vi "testWriteFileStylesheetAbsUrlHeaderPresent.vi"(8 "error in (no error)":errorcluster, 11 "TestCase in":refnum<class "EasyXMLTest.lvclass">) -> (0 "error out":errorcluster, 3 "TestCase out":refnum<class "EasyXMLTest.lvclass">)   [LabVIEW 2013, in "EasyXMLTest.lvclass"]
doc: "Verify that expected stylesheet headers are present when a stylesheet is specified"
uses:
  EasyXMLTest.lvclass
panel:
  out "XML File Header":string
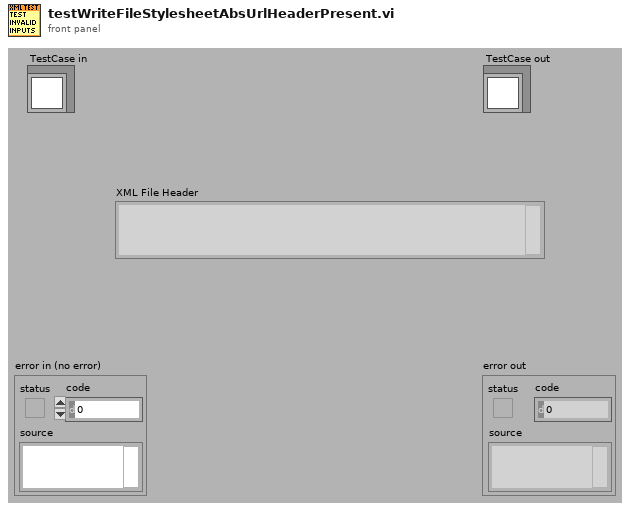
[diagram p1: front panel]
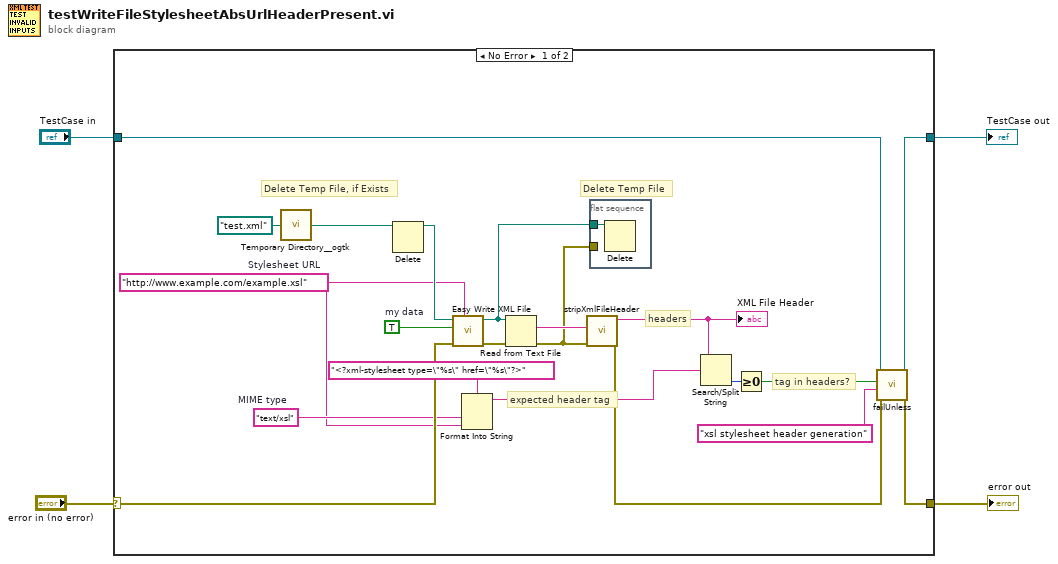
[diagram p0: block diagram]
diagram:
  n1 = case shown="No Error" "error in (no error)" {
    selector: "error in (no error)" -> [w24 w28]
    tunnel: [w11 w28] -> w3
    tunnel: [w13 w27] -> w1
    tunnel: "TestCase in" -> [w14 w27]
    frame No Error {
      w6 = "text/xsl"  # MIME type
      w5 = "http://www.example.com/example.xsl"  # Stylesheet URL
      w25 = TRUE  # my data
      # "tag in headers?"
      # "headers"
      # "expected header tag"
      # "Delete Temp File"
      # "Delete Temp File, if Exists"
      n2 = call <userlib>:"Temporary Directory__ogtk.vi"("Relative path (.)"=path "test.xml") -> ("Temporary Directory (+ Relative)"=w22:path)
      n3 = Delete(path (use dialog)=w22) -> (deleted path=w21:path)  [unwired: 4 in, 2 out]
      n4 = call "Easy Write XML File.vi"("Stylesheet URL (none)"=w5, "error in (no error)"=w24, "LabVIEW Data"=w25, "XML File Path"=w21) -> ("error out"=w19:errorcluster, "XML File Path (duplicate)"=w20:path)  [unwired: 6 in]
      n5 = Format Into String(format string="<?xml-stylesheet type=\"%s\" href=\"%s\"?>" ("Stylesheet URL (none)"), w6, w5) -> (resulting string=w7:string)  [unwired: 2 in, 1 out]
      n6 = Read from Text File(file (use dialog)=w20, error in=w19) -> (text=w18:string, error out=w17:errorcluster)  [unwired: 2 in, 2 out]
      n7 = call "stripXmlFileHeader.vi"("error in (no error)"=w17, "XML File String"=w18) -> ("error out"=w12:errorcluster, "XML File Header"=w16:string)  [unwired: 7 in, 1 out]
      "XML File Header" <- w16
      n8 = flat-sequence {
        tunnel: w20 -> [w26]
        tunnel: w17 -> [_]
        frame #0 {
          n9 = Delete(path (use dialog)=w26) -> ()  [unwired: 4 in, 3 out]
        }
      }
      n10 = Search/Split String(string=w16, search string/char (-)=w7) -> (offset of match=w15:i32)  [unwired: 1 in, 2 out]
      n11 = Greater Or Equal To 0?(x=w15) -> (x >= 0?=w10:bool)
      n12 = call-dynamic "failUnless.vi"("error in (no error)"=w12, "message (\"\")"="xsl stylesheet header generation" ("message (\"\")"), "pass"=w10, "TestCase in"=w14) -> ("error out"=w11:errorcluster, "TestCase out"=w13:refnum<class "EasyXMLTest.lvclass">)  [unwired: 6 in]
    }
    frame Error {
    }
  }
  "error out" <- w3
  "TestCase out" <- w1
